vi "EmptyTree__slk_tc.vi"(0 "tree control in":refnum<class "TreeControl.lvclass">, 1 "return elements (F)":bool, 11 "error in (no error)":errorcluster) -> (4 "tree control out":refnum<class "TreeControl.lvclass">, 6 "all elements":string[](array[string]), 15 "error out":errorcluster)   [LabVIEW 2020, in "TreeControl.lvclass"]
doc: "Deletes all elements from Tree Reference In. Passes deleted elements from the tree out in a 1-D array. The array is ordered top to bottom item as they were in the tree."
uses:
  Library/TreeControl.lvclass
  Library/TreeControl.lvclass/TreeControl.ctl
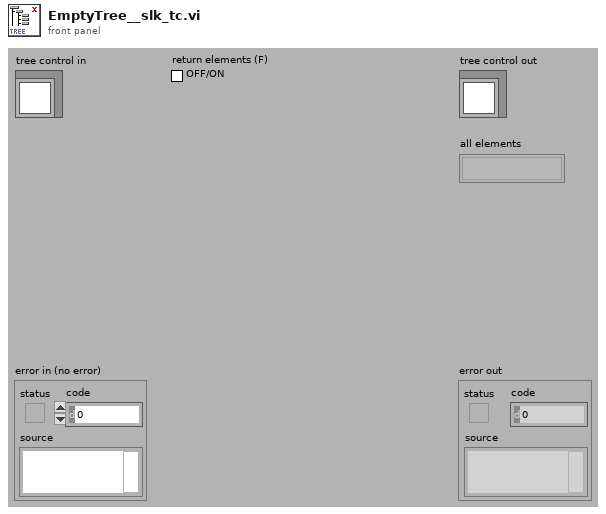
[diagram p1: front panel]
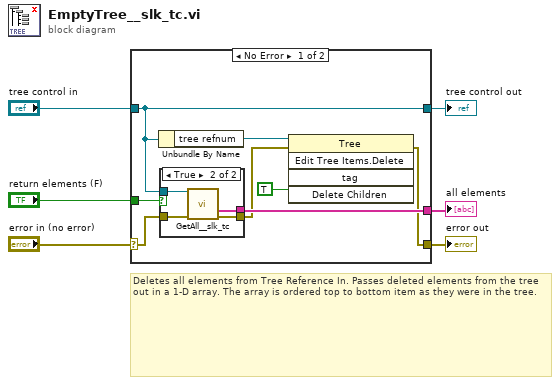
[diagram p0: block diagram]
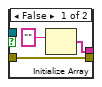
[diagram p2: hidden frame]
diagram:
  # "Deletes all elements from Tree Reference In. Passes deleted elements from the tree out in a 1-D array. The array is ordered top to bottom item as they were in the tree."
  n1 = case shown="No Error" "error in (no error)" {
    selector: "error in (no error)" -> [w8 w23]
    tunnel: [w7 w23] -> w5
    tunnel: [w13 w22] -> w3
    tunnel: "tree control in" -> [w13 w22]
    tunnel: "return elements (F)" -> [w14 _]
    tunnel: [w12 _] -> w1
    frame No Error {
      n2 = Unbundle By Name(w13) -> ("tree refnum"=w11:refnum<vi>)
      n3 = case shown="True" w14 {
        tunnel: w13 -> [_ w21]
        tunnel: w8 -> [w15 w20]
        tunnel: [w17 w19] -> w12
        tunnel: [w15 w18] -> w10
        frame False {
          n4 = Initialize Array("") -> (w17:string[])  [unwired: 1 out]
        }
        frame True {
          n5 = call "GetAll__slk_tc.vi"("tree control in"=w21, "error in (no error)"=w20) -> ("output tree items"=w19:string[], "error out"=w18:errorcluster)  [unwired: 12 out]
        }
      }
      n6 = invoke class="Tree" method="Edit Tree Items.Delete"(reference=w11, error in=w10, "Delete Children"=TRUE ("Delete Children?")) -> (error out=w7:errorcluster)  [unwired: 2 in, 4 out]
    }
    frame Error {
    }
  }
  "error out" <- w5
  "tree control out" <- w3
  "all elements" <- w1
